vi "Master Setup Read RT Update Timestamp.vi"(8 "error in (no error)":errorcluster, 10 "Pattern Label":T1 items=["Channel Setup (0)", "PID Setup (1)", "Filter Setup (2)", "~Reserved Old CAN Msgs (3)", "~Reserved Old CAN1 (4)", "~Reserved Old CAN2 (5)", "Digital Inputs Setup (6)", "Digital Outputs Setup (7)", "Logging 1 Setup (8)", "Logging 2 Setup (9)", "Logging 3 Setup (10)", "Setpoint Setup (11)", "Test Series Setup (12)", "Graph Setup (13)", "System Configure (14)", "Header (15)", "Profile Manager (16)", "Post-Mortem Logging (17)", "High-Speed Data (18)", "Statistic Channel Setup (19)", "Ramp Channel Setup (20)", "ETAS INCA Channel Setup (21)", "ETC ECCS Transducer Setup (22)", "ETC ECCS Test Setup (23)", "AVL AK Smoke Meter Setup (24)", "Triggers Setup (25)", "Alarm Limits Setup (26)", "YKWT1 Measurement (27)", "YKWT1 Instrument (28)", "Auto File Settings (29)", "Playback File Setting (30)", "UUT Constants (31)", "UPS Setup (32)", "Differential Channel Setup (33)", "Integral Channel Setup (34)", "Signal Channel Setup (35)", "Calibration Setup (36)", "BNC Setup (37)", "ASAP3 Setup (38)", "Chassis Force Calculations (39)", "Chassis Teststand Losses (40)", "Chassis Vehicle Losses (41)", "Formula Channels (42)", "ASAP3 Map Coords Setup (43)", "Digital Controls Setup (44)", "Push Buttons Setup (45)", "Sliders Setup (46)", "~Reserved~ (47)", "Email Setup (48)", "Timer Setup (49)", "Unit Conversion Setup (50)", "Visible Channels (51)", "Main Display Setup (52)", "Message Display Setup (53)", "Input Display Setup (54)", "Unico Parameter Downloads (55)", "Flow Meter Setup (56)", "Channel Zero Offset (57)", "YKWT2 Measurement (58)", "YKWT2 Instrument (59)", "~Reserved Old CAN3 (60)", "CAS Setup (61)", "Accumulation Channel Setup (62)", "Valvetrain Dynamics Setup (63)", "CCP Setup (64)", "System Log Setup (65)", "Throttle Controller (66)", "RE Shifter (67)", "Main Display (68)", "~Reserved~ (69)", "FlexRay (70)", "YKWT3 Measurement (71)", "YKWT3 Instrument (72)", "CAN XNET API (73)"]) -> (0 "error out":errorcluster, 3 "RT Setup String (out)":timestamp)   [LabVIEW 2017]
uses:
  Master Setup Pattern Enum.ctl
panel:
  in  "Setup File (System Configure)":path=path "C:/Revolutionary Engineering/REPS/Setup Files/Default/GM Trans Cell 2/SystemConfigure GM cell 2.cfs"
  in  "Setup File (Setpoint)":path=path "C:/Revolutionary Engineering/REPS/Setup Files/Default/RE Cell 3-1/re cell 3 setpoints.spt"
  in  "Setup File (CAN 0)":path
  in  "Setup File (CAN 1)":path
  in  "Setup File (Can Message)":path
  in  "Setup File (Playback)":path
  in  "Setup File (UUT Constants)":path
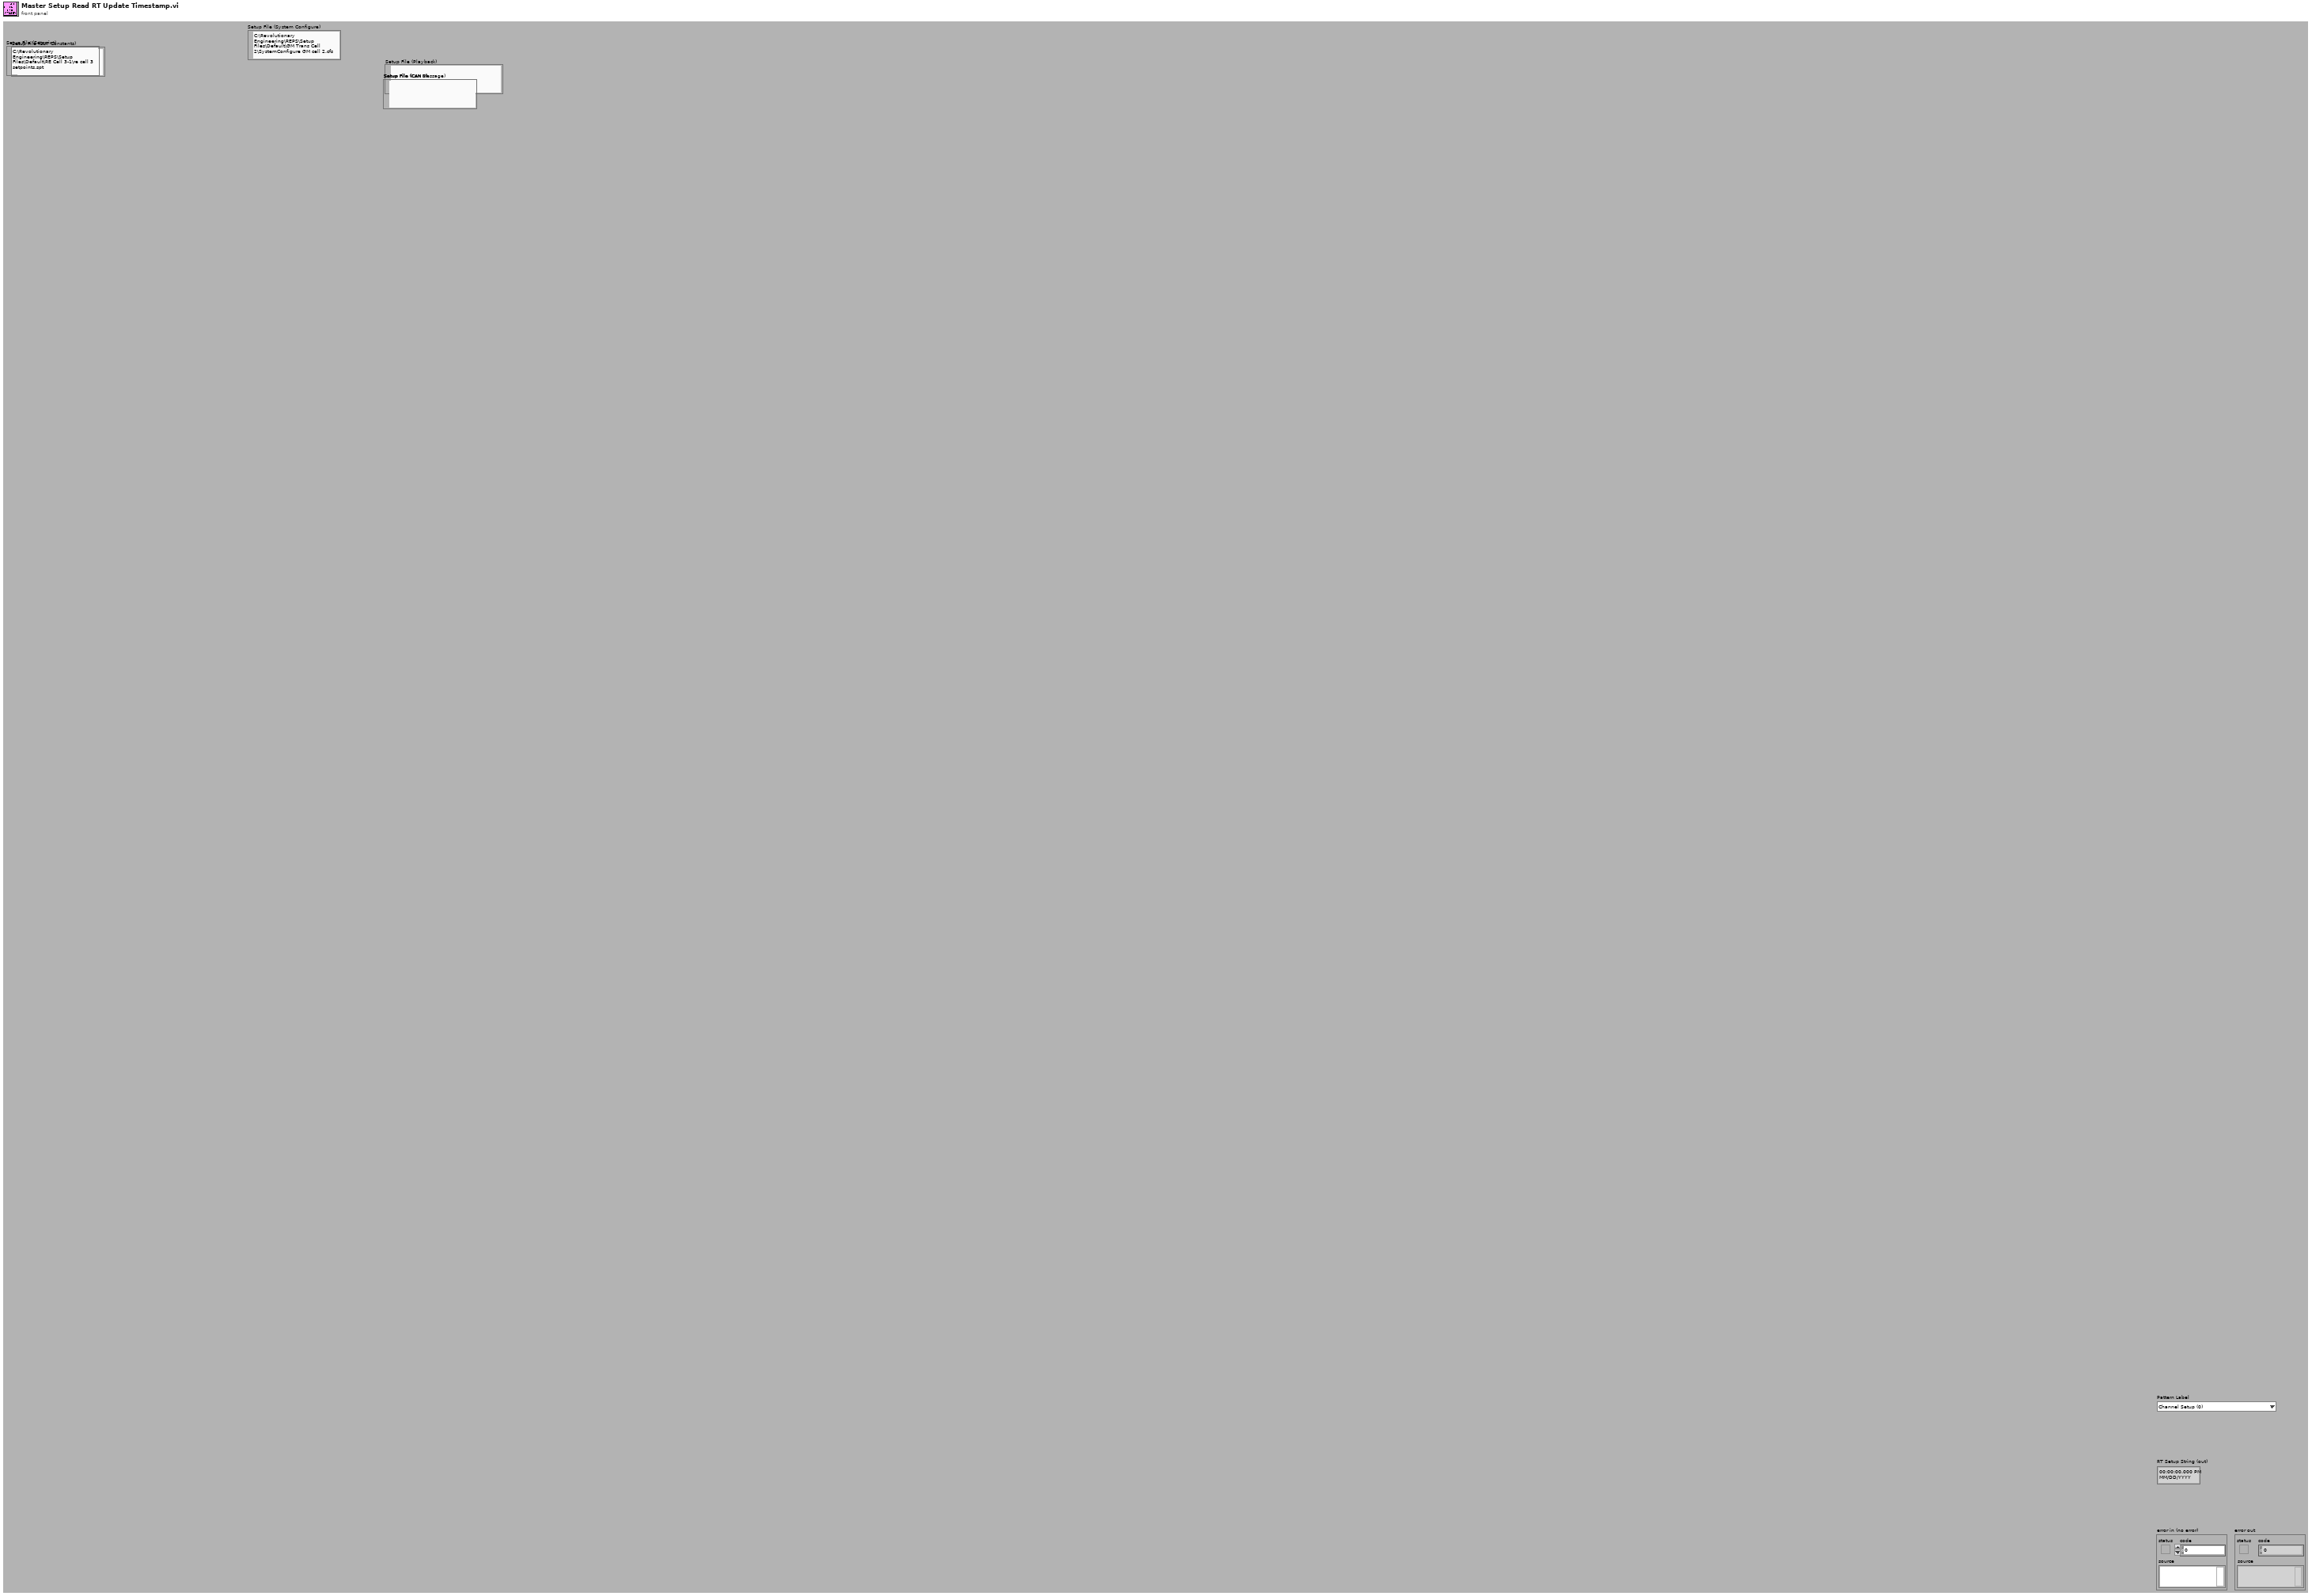
[diagram p1: front panel]
types:
  T1 = typedef "Master Setup Pattern Enum.ctl" = i32
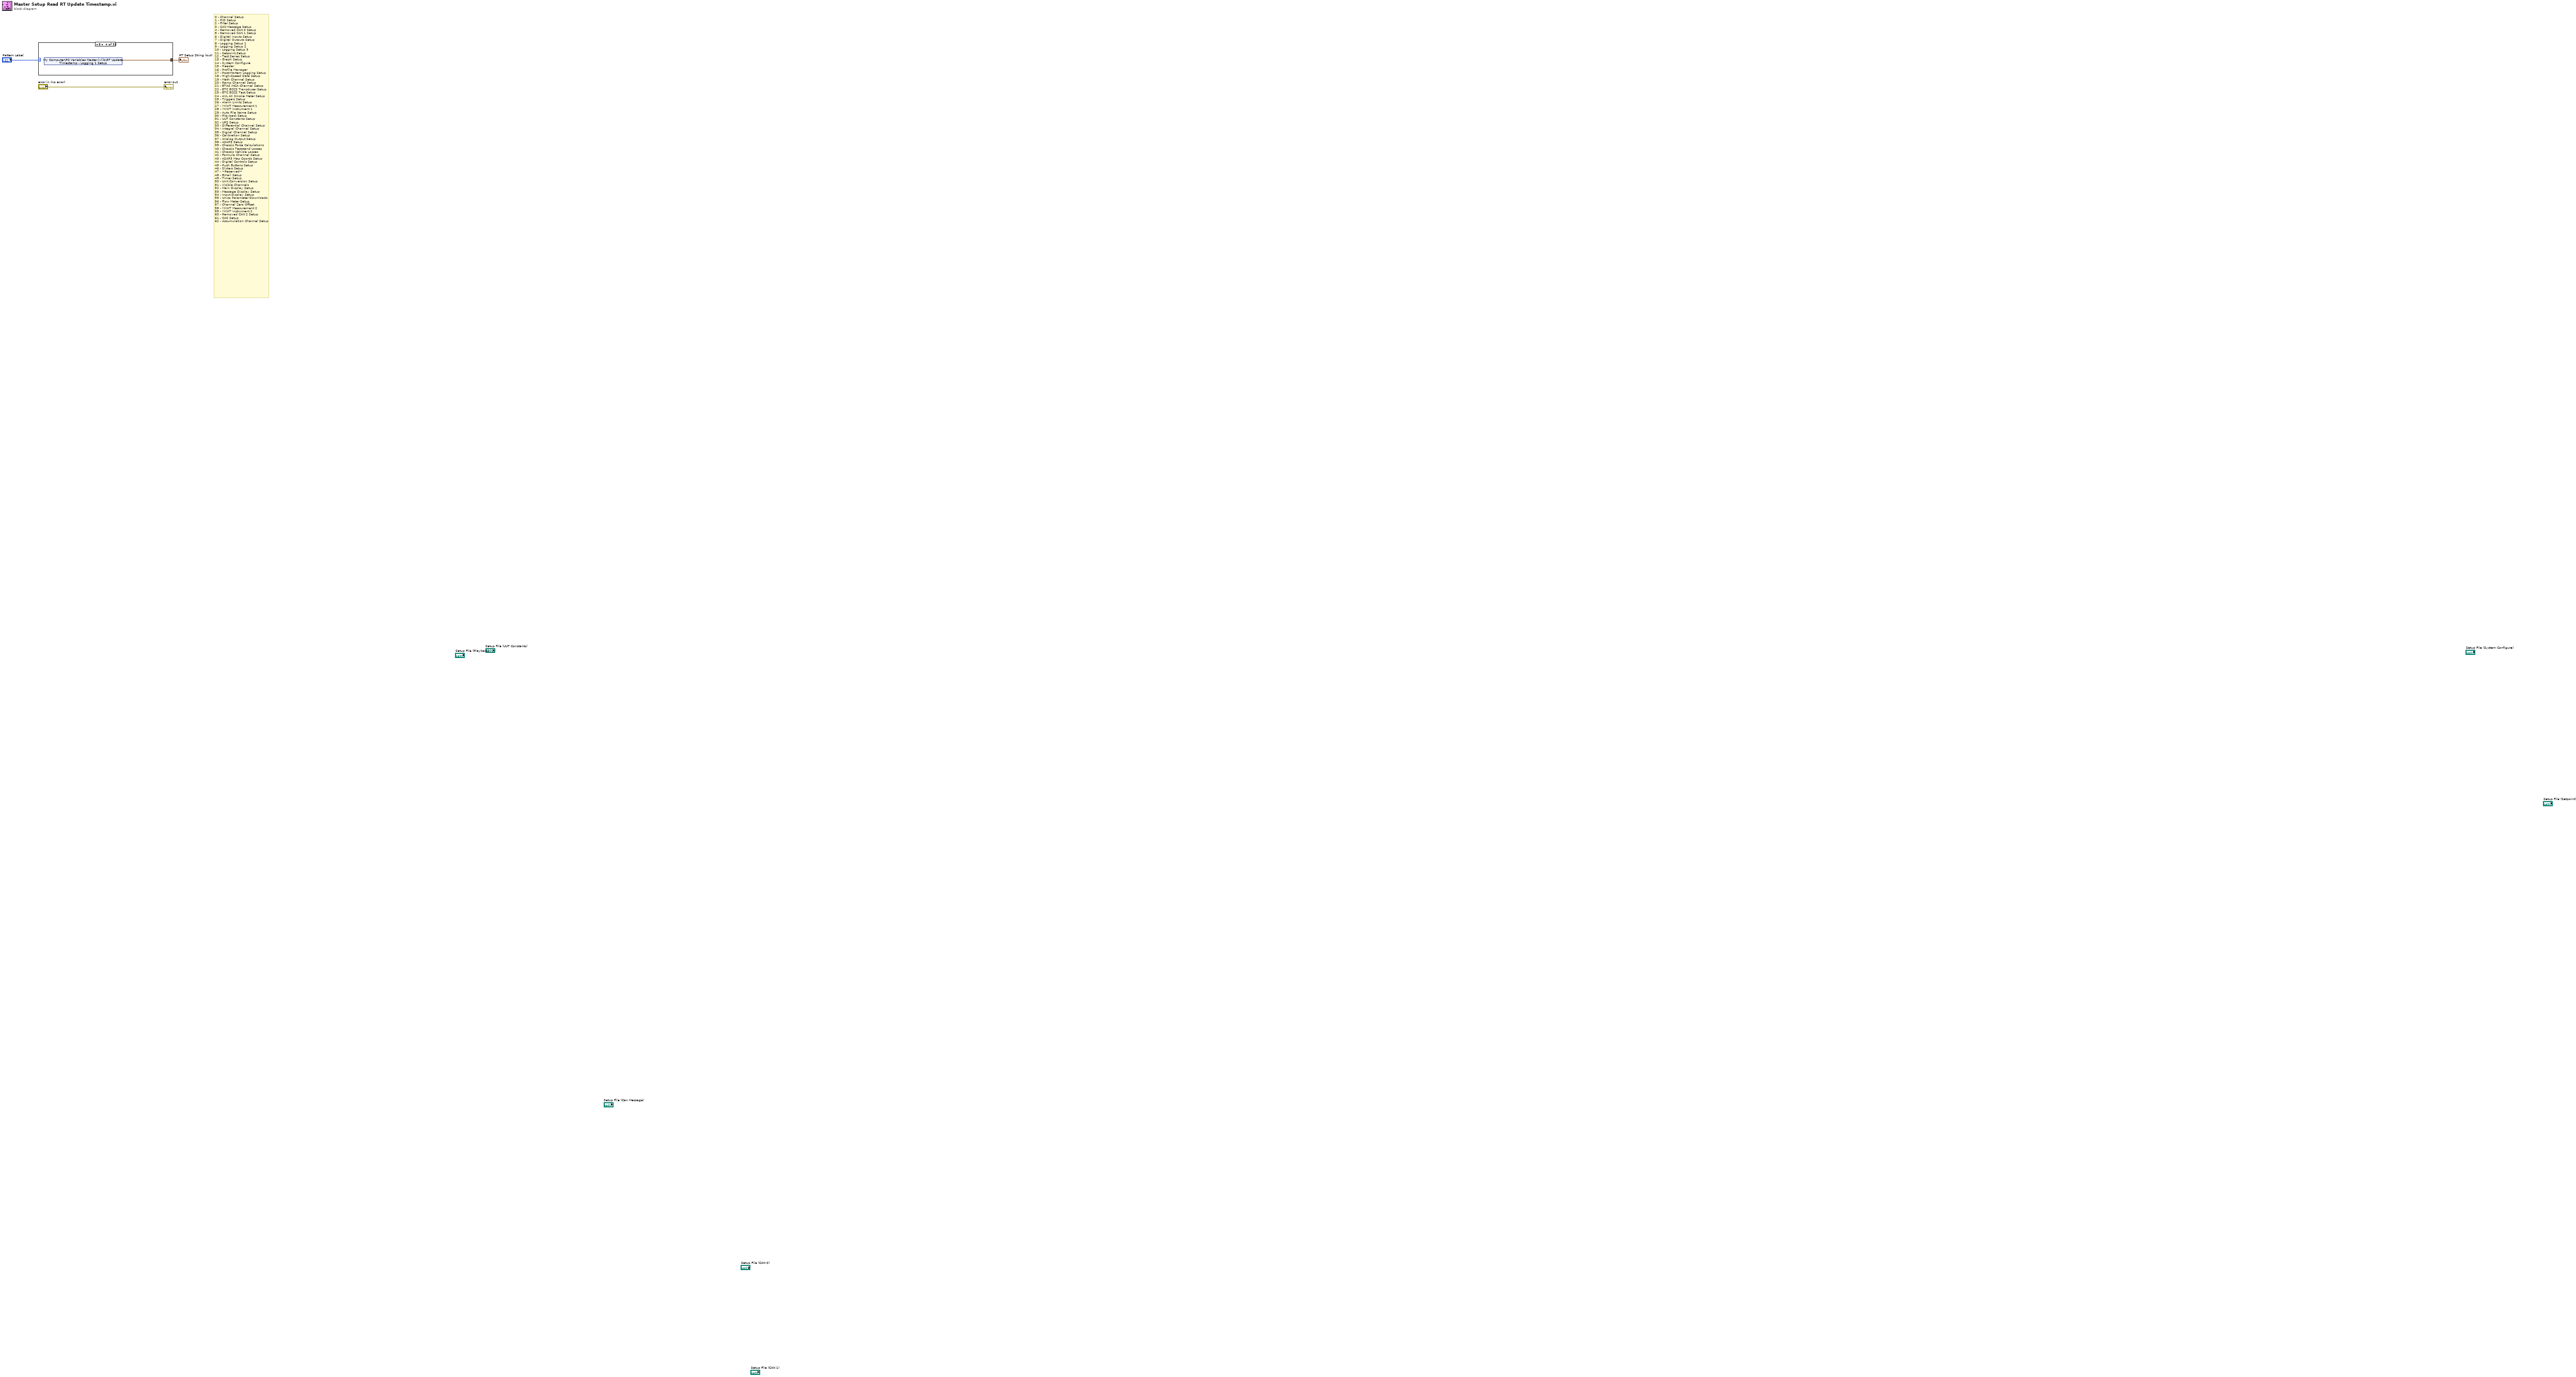
[diagram p0: block diagram]
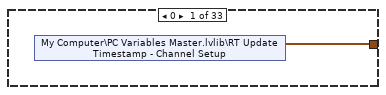
[diagram p2: hidden frame]
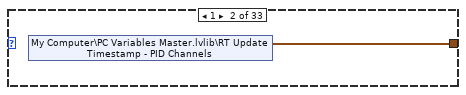
[diagram p3: hidden frame]
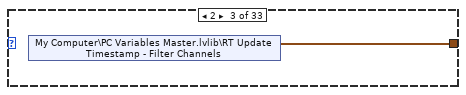
[diagram p4: hidden frame]
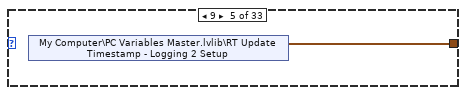
[diagram p5: hidden frame]
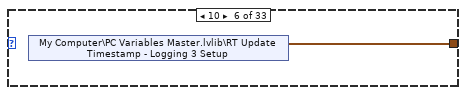
[diagram p6: hidden frame]
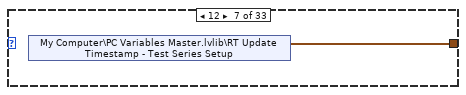
[diagram p7: hidden frame]
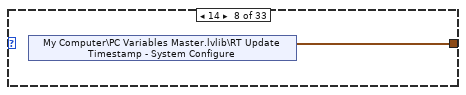
[diagram p8: hidden frame]
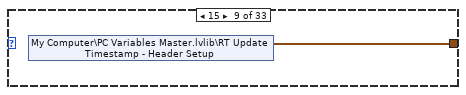
[diagram p9: hidden frame]
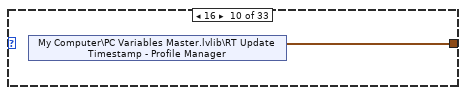
[diagram p10: hidden frame]
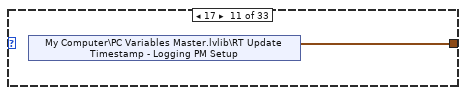
[diagram p11: hidden frame]
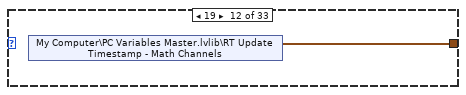
[diagram p12: hidden frame]
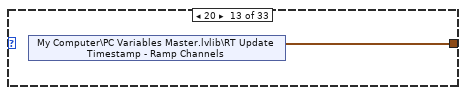
[diagram p13: hidden frame]
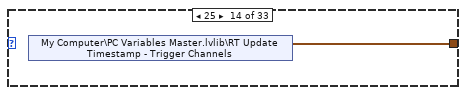
[diagram p14: hidden frame]
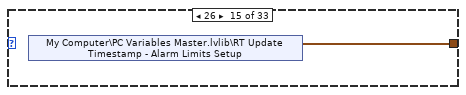
[diagram p15: hidden frame]
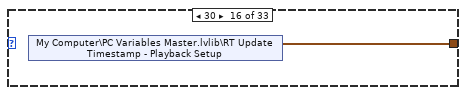
[diagram p16: hidden frame]
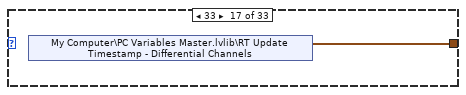
[diagram p17: hidden frame]
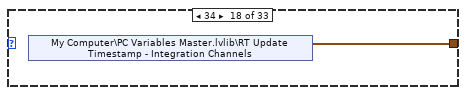
[diagram p18: hidden frame]
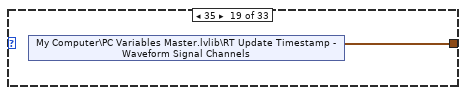
[diagram p19: hidden frame]
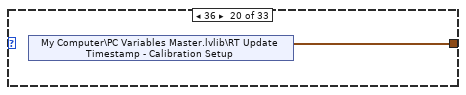
[diagram p20: hidden frame]
diagram:
  # "0 - Channel Setup\n1 - PID Setup\n2 - Filter Setup\n3 - CAN Message Setup\n4 - Removed CAN 0 Setup\n5 - Removed CAN 1 Setup\n6 - Digital Inputs Setup\n7 - Digital Outputs Setup\n8 - Logging Setup 1\n9 - Logging Setup 2\n10 - Logging Setup 3\n11 - Setpoint Setup\n12 - Test Series Setup\n13 - Graph Setup\n14 - System Configure\n15 - Header\n16 - Profile Manager\n17 - Post-Mortem Logging Setup\n18 - High-Speed Data Setup\n19 - Math Channel Setup\n20 - Ramp Channel Setup\n21 - ETAS INCA Channel Setup\n22 - ETC ECCS Transducer Setup\n23 - ETC ECCS Test Setup\n24 - AVL AK Smoke Meter Setup\n25 - Triggers Setup\n26 - Alarm Limits Setup\n27 - YKWT Measurement 1\n28 - YKWT Instrument 1\n29 - Auto File Name Setup\n30 - Playback Setup\n31 - UUT Constants Setup\n32 - UPS Setup\n33 - Differential Channel Setup\n34 - Integral Channel Setup\n35 - Signal Channel Setup\n36 - Calibration Setup\n37 - Analog Output Setup\n38 - ASAP3 Setup\n39 - Chassis Force Calculations\n40 - Chassis Teststand Losses\n41 - Chassis Vehicle Losses\n42 - Formula Channel Setup\n43 - ASAP3 Map Coords Setup\n44 - Digital Controls Setup\n45 - Push Buttons Setup\n46 - Sliders Setup\n47 - ~Reserved~\n48 - Email Setup\n49 - Timer Setup\n50 - Unit Conversion Setup\n51 - Visible Channels\n52 - Main Display Setup\n53 - Message Display Setup\n54 - Input Display Setup\n55 - Unico Parameter Downloads\n56 - Flow Meter Setup\n57 - Channel Zero Offset\n58 - YKWT Measurement 2\n59 - YKWT Instrument 2\n60 - Removed CAN 2 Setup\n61 - CAS Setup\n62 - Accumulation Channel Setup"
  n1 = case shown="8" "Pattern Label" {
    tunnel: [w4 w5 w6 w7 w8 w9 w10 w11 w12 w13 w14 w15 w16 w17 w18 w19 w20 w21 w22 w23 w24 w25 w26 w27 w28 w29 w30 w31 w32 w33 w34 w35 timestamp(0 s since 1904-01-01) ("Timestamp")] -> w1
    frame 0 {
      n2 = shared-variable "My Computer\\PC Variables Master.lvlib\\RT Update Timestamp - Channel Setup"() -> (w4:timestamp)  [unwired: 1 in, 1 out]
    }
    frame 1 {
      n3 = shared-variable "My Computer\\PC Variables Master.lvlib\\RT Update Timestamp - PID Channels"() -> (w5:timestamp)  [unwired: 1 in, 1 out]
    }
    frame 2 {
      n4 = shared-variable "My Computer\\PC Variables Master.lvlib\\RT Update Timestamp - Filter Channels"() -> (w6:timestamp)  [unwired: 1 in, 1 out]
    }
    frame 8 {
      n5 = shared-variable "My Computer\\PC Variables Master.lvlib\\RT Update Timestamp - Logging 1 Setup"() -> (w7:timestamp)  [unwired: 1 in, 1 out]
    }
    frame 9 {
      n6 = shared-variable "My Computer\\PC Variables Master.lvlib\\RT Update Timestamp - Logging 2 Setup"() -> (w8:timestamp)  [unwired: 1 in, 1 out]
    }
    frame 10 {
      n7 = shared-variable "My Computer\\PC Variables Master.lvlib\\RT Update Timestamp - Logging 3 Setup"() -> (w9:timestamp)  [unwired: 1 in, 1 out]
    }
    frame 12 {
      n8 = shared-variable "My Computer\\PC Variables Master.lvlib\\RT Update Timestamp - Test Series Setup"() -> (w10:timestamp)  [unwired: 1 in, 1 out]
    }
    frame 14 {
      n9 = shared-variable "My Computer\\PC Variables Master.lvlib\\RT Update Timestamp - System Configure"() -> (w11:timestamp)  [unwired: 1 in, 1 out]
    }
    frame 15 {
      n10 = shared-variable "My Computer\\PC Variables Master.lvlib\\RT Update Timestamp - Header Setup"() -> (w12:timestamp)  [unwired: 1 in, 1 out]
    }
    frame 16 {
      n11 = shared-variable "My Computer\\PC Variables Master.lvlib\\RT Update Timestamp - Profile Manager"() -> (w13:timestamp)  [unwired: 1 in, 1 out]
    }
    frame 17 {
      n12 = shared-variable "My Computer\\PC Variables Master.lvlib\\RT Update Timestamp - Logging PM Setup"() -> (w14:timestamp)  [unwired: 1 in, 1 out]
    }
    frame 19 {
      n13 = shared-variable "My Computer\\PC Variables Master.lvlib\\RT Update Timestamp - Math Channels"() -> (w15:timestamp)  [unwired: 1 in, 1 out]
    }
    frame 20 {
      n14 = shared-variable "My Computer\\PC Variables Master.lvlib\\RT Update Timestamp - Ramp Channels"() -> (w16:timestamp)  [unwired: 1 in, 1 out]
    }
    frame 25 {
      n15 = shared-variable "My Computer\\PC Variables Master.lvlib\\RT Update Timestamp - Trigger Channels"() -> (w17:timestamp)  [unwired: 1 in, 1 out]
    }
    frame 26 {
      n16 = shared-variable "My Computer\\PC Variables Master.lvlib\\RT Update Timestamp - Alarm Limits Setup"() -> (w18:timestamp)  [unwired: 1 in, 1 out]
    }
    frame 30 {
      n17 = shared-variable "My Computer\\PC Variables Master.lvlib\\RT Update Timestamp - Playback Setup"() -> (w19:timestamp)  [unwired: 1 in, 1 out]
    }
    frame 33 {
      n18 = shared-variable "My Computer\\PC Variables Master.lvlib\\RT Update Timestamp - Differential Channels"() -> (w20:timestamp)  [unwired: 1 in, 1 out]
    }
    frame 34 {
      n19 = shared-variable "My Computer\\PC Variables Master.lvlib\\RT Update Timestamp - Integration Channels"() -> (w21:timestamp)  [unwired: 1 in, 1 out]
    }
    frame 35 {
      n20 = shared-variable "My Computer\\PC Variables Master.lvlib\\RT Update Timestamp - Waveform Signal Channels"() -> (w22:timestamp)  [unwired: 1 in, 1 out]
    }
    frame 36 {
      n21 = shared-variable "My Computer\\PC Variables Master.lvlib\\RT Update Timestamp - Calibration Setup"() -> (w23:timestamp)  [unwired: 1 in, 1 out]
    }
    frame 37 {
      n22 = shared-variable "My Computer\\PC Variables Master.lvlib\\RT Update Timestamp - BNC Setup"() -> (w24:timestamp)  [unwired: 1 in, 1 out]
    }
    frame 42 {
      n23 = shared-variable "My Computer\\PC Variables Master.lvlib\\RT Update Timestamp - Formula Channels"() -> (w25:timestamp)  [unwired: 1 in, 1 out]
    }
    frame 45 {
      n24 = shared-variable "My Computer\\PC Variables Master.lvlib\\RT Update Timestamp - Push Button Setup"() -> (w26:timestamp)  [unwired: 1 in, 1 out]
    }
    frame 49 {
      n25 = shared-variable "My Computer\\PC Variables Master.lvlib\\RT Update Timestamp - Timer Channels"() -> (w27:timestamp)  [unwired: 1 in, 1 out]
    }
    frame 50 {
      n26 = shared-variable "My Computer\\PC Variables Master.lvlib\\RT Update Timestamp - Unit Conversion"() -> (w28:timestamp)  [unwired: 1 in, 1 out]
    }
    frame 56 {
      n27 = shared-variable "My Computer\\PC Variables Master.lvlib\\RT Update Timestamp - Flow Meter Channels"() -> (w29:timestamp)  [unwired: 1 in, 1 out]
    }
    frame 57 {
      n28 = shared-variable "My Computer\\PC Variables Master.lvlib\\RT Update Timestamp - Zero Offset Setup"() -> (w30:timestamp)  [unwired: 1 in, 1 out]
    }
    frame 62 {
      n29 = shared-variable "My Computer\\PC Variables Master.lvlib\\RT Update Timestamp - Accumulation Channels"() -> (w31:timestamp)  [unwired: 1 in, 1 out]
    }
    frame 65 {
      n30 = shared-variable "My Computer\\PC Variables Master.lvlib\\RT Update Timestamp - System Log"() -> (w32:timestamp)  [unwired: 1 in, 1 out]
    }
    frame 64 {
      n31 = shared-variable "My Computer\\PC Variables Master.lvlib\\RT Update Timestamp - CCP"() -> (w33:timestamp)  [unwired: 1 in, 1 out]
    }
    frame 70 {
      n32 = shared-variable "My Computer\\PC Variables Master.lvlib\\RT Update Timestamp - FlexRay"() -> (w34:timestamp)  [unwired: 1 in, 1 out]
    }
    frame 73 {
      n33 = shared-variable "My Computer\\PC Variables Master.lvlib\\RT Update Timestamp - CAN XNET API"() -> (w35:timestamp)  [unwired: 1 in, 1 out]
    }
    frame Default {
    }
  }
  "RT Setup String (out)" <- w1
  "error out" <- "error in (no error)"
